vi "GenericIMAQGetInterface.vi"(10 "Settings":T1={"Framerate (Hz)"=60, "Exposure time (us)"=5000, "Image size"={"Width"=1280, "Height"=1024}, "Number of buffers"=30}, 11 "IMAQ Camera serial config":T10={"Use serial commands directly"=FALSE, "Frame rate set cmd"="ssf %d", "Exposure time set cmd"="set %d", "Frame rate get cmd"="get ssf", "Exposure time get cmd"="get set", "IMAQ Identifier"="img0", "Serial return skip chars"=2, "Set width/height"="get set", "Set offset xy"="get set", "Get width"="get set", "Get height"="get set", "Get offset X"="get set", "Get offset Y"="get set", "Full frame size"={"width"=0, "height"=0}}) -> (3 "Camera state":T2)   [LabVIEW 2011]
uses:
  GenericIMAQHardwareConfig.ctl
  Main/Camera/CameraInstance.ctl
  CameraInterface/CameraInterface.ctl
  CameraInterface/CICloseType.ctl
  CameraInterface/CIGetSetGenericConfig.ctl
  CameraInterface/CIGrabType.ctl
  CameraInterface/CISettingsDlg.ctl
  CameraInterface/CIAdjustBeadPos.ctl
  CameraInterface/CISaveLoadSettings.ctl
  Main/Camera/GenericCameraConfigType.ctl
  GenericIMAQCameraInstance.ctl
  Global_GenericIMAQCamera_HardwareConfig.vi
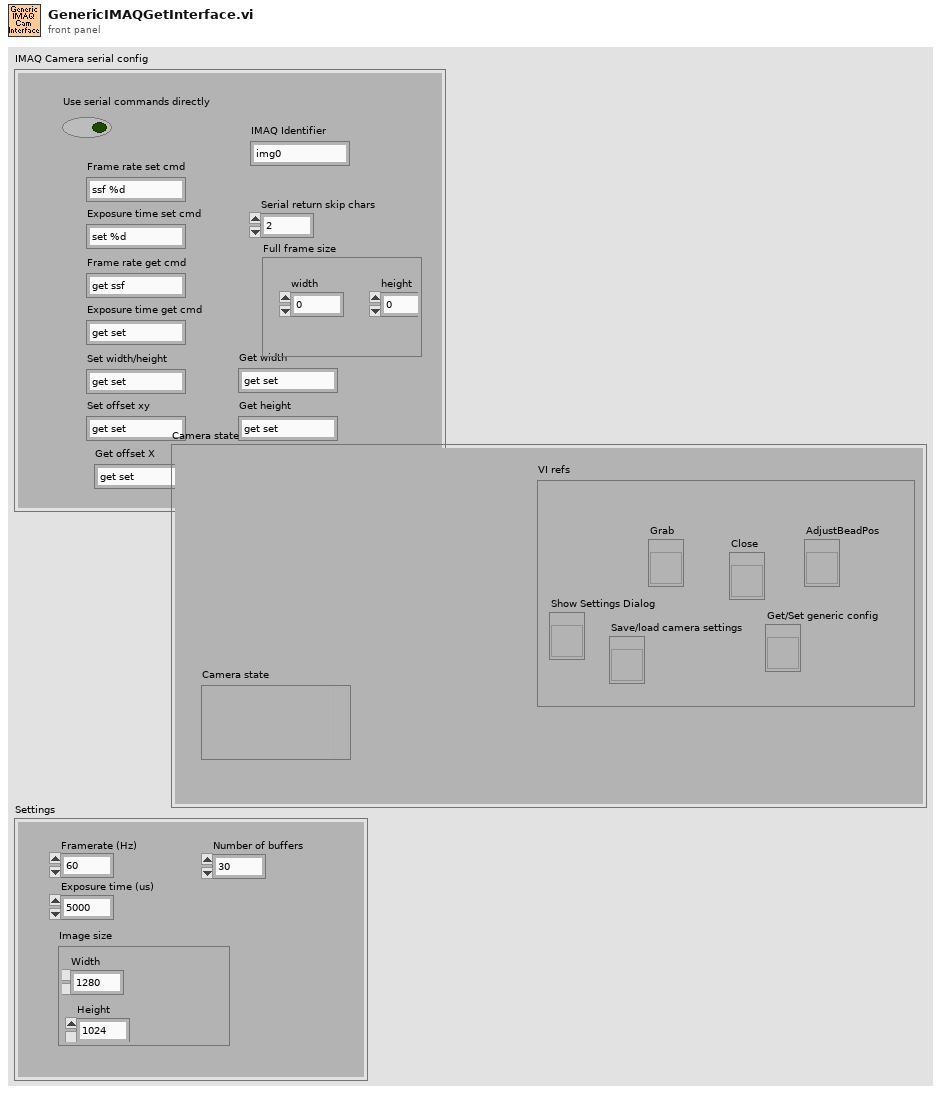
[diagram p1: front panel]
types:
  T1 = typedef "GenericCameraConfigType.ctl" = cluster{"Framerate (Hz)":i32, "Exposure time (us)":i32, "Image size":cluster{"Width":i32, "Height":i32}, "Number of buffers":i32}
  T2 = typedef "CameraInstance.ctl" = cluster{"VI refs":T3, "Camera state":variant}
  T3 = typedef "CameraInterface.ctl" = cluster{"Close":T4, "Get/Set generic config":T5, "Grab":T6, "Show Settings Dialog":T7, "AdjustBeadPos":T8, "Save/load camera settings":T9}
  T4 = typedef "CICloseType.ctl" = refnum<vi>
  T5 = typedef "CIGetSetGenericConfig.ctl" = refnum<vi>
  T6 = typedef "CIGrabType.ctl" = refnum<vi>
  T7 = typedef "CISettingsDlg.ctl" = refnum<vi>
  T8 = typedef "CIAdjustBeadPos.ctl" = refnum<vi>
  T9 = typedef "CISaveLoadSettings.ctl" = refnum<vi>
  T10 = typedef "GenericIMAQHardwareConfig.ctl" = cluster{"Use serial commands directly":bool, "Frame rate set cmd":string, "Exposure time set cmd":string, "Frame rate get cmd":string, "Exposure time get cmd":string, "IMAQ Identifier":string, "Serial return skip chars":i32, "Set width/height":string, "Set offset xy":string, "Get width":string, "Get height":string, "Get offset X":string, "Get offset Y":string, "Full frame size":cluster{"width":i32, "height":i32}}
  T11 = typedef "GenericIMAQCameraInstance.ctl" = cluster{"Session":refnum<k11>, "Settings":T1}
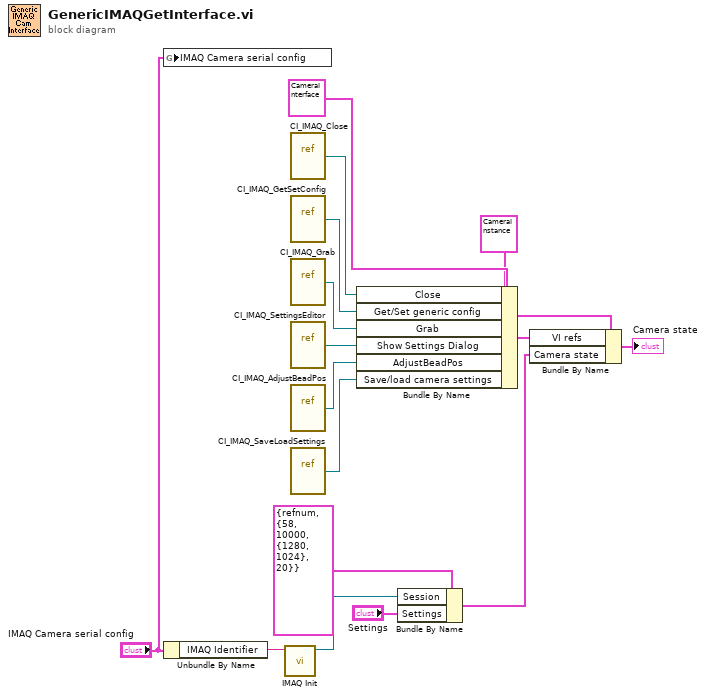
[diagram p0: block diagram]
diagram:
  n1 = global write "Global_GenericIMAQCamera_HardwareConfig.vi" "IMAQ Camera serial config"("IMAQ Camera serial config") -> ()
  n2 = Unbundle By Name("IMAQ Camera serial config") -> ("IMAQ Identifier"=w5:string)
  n3 = call <vilib>:"IMAQ Init.vi"("Interface Name"=w5) -> ("IMAQ Session Out"=w1:refnum<k11>)  [unwired: 9 in, 1 out]
  n4 = vi-ref "CI_IMAQ_Close.vi"() -> (w15:refnum<vi>)
  n5 = vi-ref "CI_IMAQ_GetSetConfig.vi"() -> (w14:refnum<vi>)
  n6 = vi-ref "CI_IMAQ_Grab.vi"() -> (w11:refnum<vi>)
  n7 = vi-ref "CI_IMAQ_SettingsEditor.vi"() -> (w12:refnum<vi>)
  n8 = vi-ref "CI_IMAQ_AdjustBeadPos.vi"() -> (w13:refnum<vi>)
  n9 = vi-ref "CI_IMAQ_SaveLoadSettings.vi"() -> (w10:refnum<vi>)
  n10 = Bundle By Name(cluster=T3 {"Close"=refnum, "Get/Set generic config"=refnum, "Grab"=refnum, "Show Settings Dialog"=refnum, "AdjustBeadPos"=refnum, "Save/load camera settings"=refnum} ("Camera interface"), "Close"=w15, "Get/Set generic config"=w14, "Grab"=w11, "Show Settings Dialog"=w12, "AdjustBeadPos"=w13, "Save/load camera settings"=w10) -> (w8:T3)
  n11 = Bundle By Name(cluster=T11 {"Session"=refnum, "Settings"={"Framerate (Hz)"=58, "Exposure time (us)"=10000, "Image size"={"Width"=1280, "Height"=1024}, "Number of buffers"=20}} ("Generic IMAQ Camera Instance"), "Session"=w1, "Settings"="Settings") -> (w3:T11)
  n12 = Bundle By Name(cluster=T2 {"VI refs"={"Close"=refnum, "Get/Set generic config"=refnum, "Grab"=refnum, "Show Settings Dialog"=refnum, "AdjustBeadPos"=refnum, "Save/load camera settings"=refnum}, "Camera state"=variant} ("Camera Instance"), "VI refs"=w8, "Camera state"=w3) -> (→"Camera state":T2)
